vi "findKingLocation.vi"() -> (0 "bj":i32, 1 "bi":i32, 2 "rj":i32, 3 "ri":i32)   [LabVIEW 2024]
uses:
  GlobalVar.vi
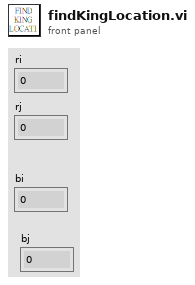
[diagram p1: front panel]
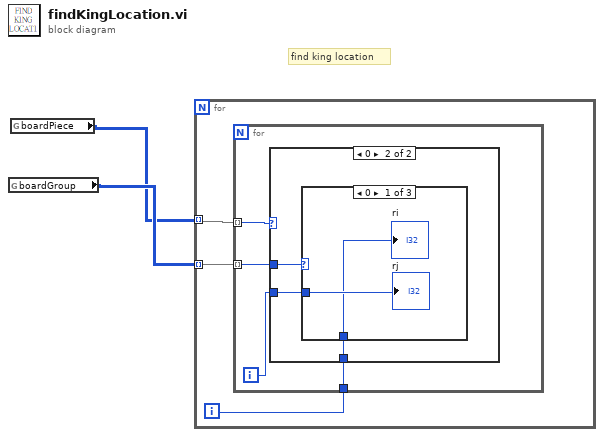
[diagram p0: block diagram]
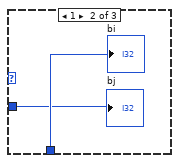
[diagram p3: hidden frame]
diagram:
  # "find king location"
  n1 = global read "GlobalVar.vi" "boardGroup"() -> (w2:i32[][])
  n2 = global read "GlobalVar.vi" "boardPiece"() -> (w1:i32[][])
  n3 = for {
    tunnel: w1 -> [w5] mode=indexing
    tunnel: w2 -> [w4] mode=indexing
    i -> [w3]
    n4 = for {
      tunnel: w5 -> [w9] mode=indexing
      tunnel: w4 -> [w8] mode=indexing
      tunnel: w3 -> [w6]
      i -> [w7]
      n5 = case shown="0" w9 {
        tunnel: w8 -> [_ w12]
        tunnel: w7 -> [_ w11]
        tunnel: w6 -> [_ w10]
        frame Default {
        }
        frame 0 {
          n6 = case shown="0" w12 {
            tunnel: w11 -> [w14 w15 _]
            tunnel: w10 -> [w13 w16 _]
            frame 0 {
              "rj" <- w14
              "ri" <- w13
            }
            frame 1 {
              "bi" <- w16
              "bj" <- w15
            }
            frame Default {
            }
          }
        }
      }
    }
  }
